vi "find_STOP.vi"(11 "Path":path) -> (0 "Y 2":sgl, 1 "X 2":sgl, 2 "Y":sgl, 3 "X":sgl)   [LabVIEW 2015]
panel:
  out "Image Out":T1(plugin-control)
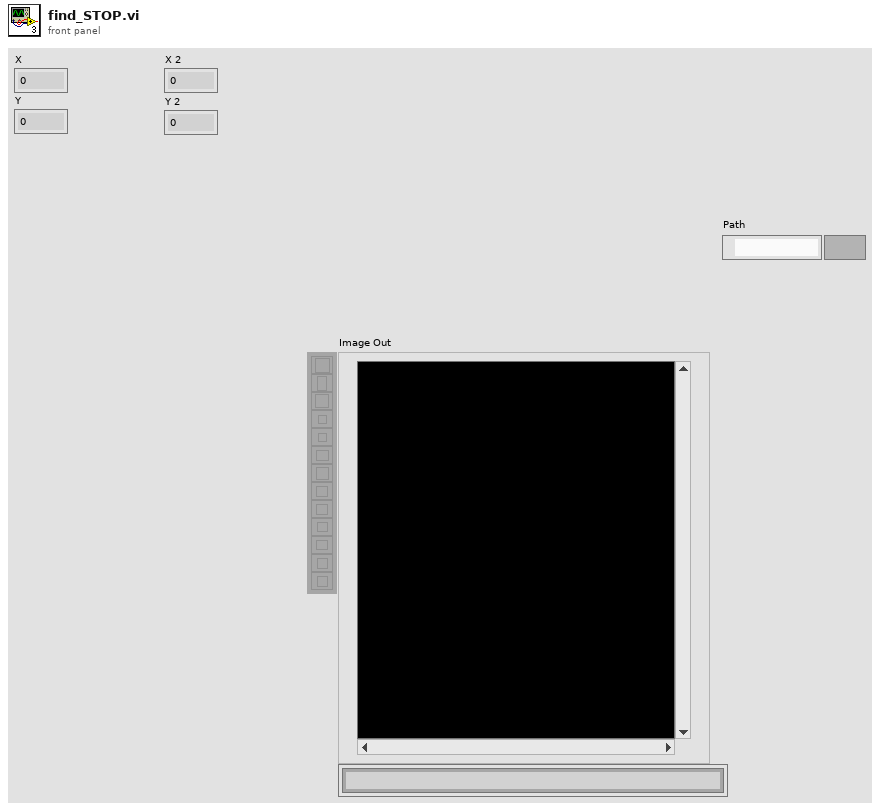
[diagram p1: front panel]
types:
  T1 = typedef "IMAQ Image.ctl" = refnum<image>
  T2 = cluster{"Corners":cluster{"X":sgl, "Y":sgl}[], "Orientation (degrees)":dbl, "Width":dbl, "Height":dbl, "Score":dbl}[]
  T3 = cluster{"Corners":cluster{"X":sgl, "Y":sgl}[], "Orientation (degrees)":dbl, "Width":dbl, "Height":dbl, "Score":dbl}
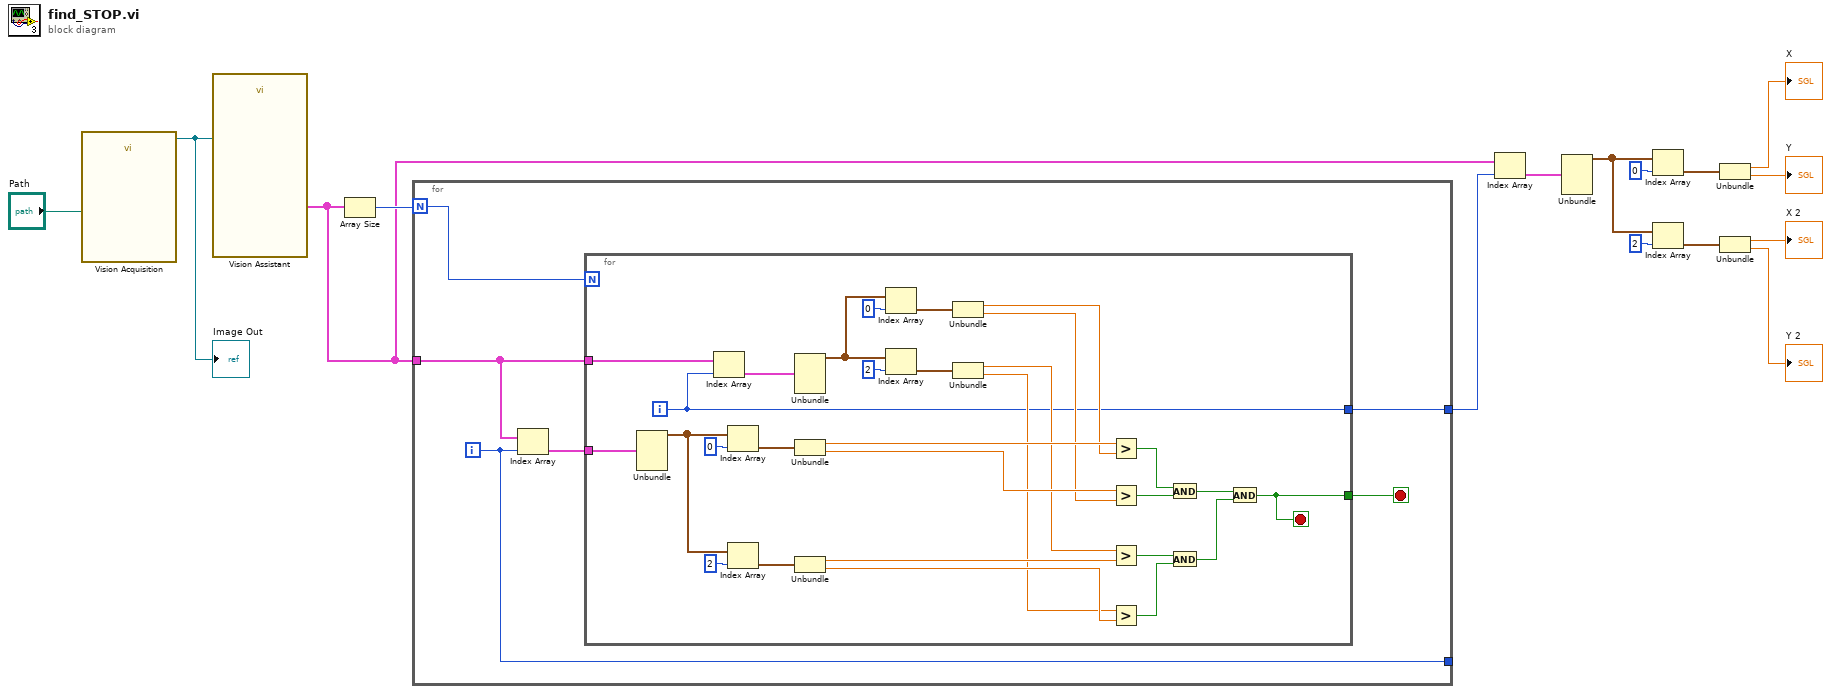
[diagram p0: block diagram]
diagram:
  n1 = call "Vision Acquisition"("Image Path"="Path") -> ("Image Out"=w11:T1)  [unwired: 25 in, 1 out]
  "Image Out" <- w11
  n2 = call "Vision Assistant"("Image In"=w11) -> ("Rectangles (Shape Detection 1)"=w13:T2)  [unwired: 23 in, 3 out]
  n3 = Array Size(array=w13) -> (size(s)=w15:i32)
  n4 = for {
    N: w15 -> [w21]
    tunnel: w13 -> [w20]
    tunnel: [w18] -> _
    tunnel: [w17] -> w14
    i -> [w18]
    stop <- w16 stop-if-true
    n5 = Index Array(array=w20, index=w18) -> (element=w19:T3)
    n6 = for {
      N: w21 -> [_]
      tunnel: w20 -> [w50]
      tunnel: w19 -> [w47]
      tunnel: [w23] -> w17
      tunnel: [w22] -> w16
      i -> [w23]
      stop <- w22 stop-if-true
      n7 = Unbundle(w47) -> ("Corners"=w39:cluster{"X":sgl, "Y":sgl}[])  [unwired: 4 out]
      n8 = Index Array(array=w50, index=w23) -> (element=w46:T3)
      n9 = Index Array(array=w39, index=0) -> (element=w49:cluster{"X":sgl, "Y":sgl})
      n10 = Index Array(array=w39, index=2) -> (element=w45:cluster{"X":sgl, "Y":sgl})
      n11 = Unbundle(w46) -> ("Corners"=w38:cluster{"X":sgl, "Y":sgl}[])  [unwired: 4 out]
      n12 = Unbundle(w49) -> ("X"=w37:sgl, "Y"=w35:sgl)
      n13 = Unbundle(w45) -> ("X"=w29:sgl, "Y"=w27:sgl)
      n14 = Index Array(array=w38, index=0) -> (element=w43:cluster{"X":sgl, "Y":sgl})
      n15 = Index Array(array=w38, index=2) -> (element=w41:cluster{"X":sgl, "Y":sgl})
      n16 = Unbundle(w43) -> ("X"=w36:sgl, "Y"=w34:sgl)
      n17 = Unbundle(w41) -> ("X"=w28:sgl, "Y"=w26:sgl)
      n18 = Greater?(x=w37, y=w36) -> (0:w33:bool)
      n19 = Greater?(x=w35, y=w34) -> (0:w32:bool)
      n20 = Greater?(x=w28, y=w29) -> (0:w31:bool)
      n21 = Greater?(x=w26, y=w27) -> (0:w30:bool)
      n22 = And(x=w33, y=w32) -> (x .and. y?=w25:bool)
      n23 = And(x=w31, y=w30) -> (x .and. y?=w24:bool)
      n24 = And(x=w25, y=w24) -> (x .and. y?=w22:bool)
    }
  }
  n25 = Index Array(array=w13, index=w14) -> (element=w10:T3)
  n26 = Unbundle(w10) -> ("Corners"=w5:cluster{"X":sgl, "Y":sgl}[])  [unwired: 4 out]
  n27 = Index Array(array=w5, index=0) -> (element=w9:cluster{"X":sgl, "Y":sgl})
  n28 = Index Array(array=w5, index=2) -> (element=w7:cluster{"X":sgl, "Y":sgl})
  n29 = Unbundle(w9) -> ("X"=→"X":sgl, "Y"=→"Y":sgl)
  n30 = Unbundle(w7) -> ("X"=→"X 2":sgl, "Y"=→"Y 2":sgl)
